vi "2013_02_18 Quality Main.vi"() -> ()   [LabVIEW 2013]
uses:
  Quality Type Def.ctl
  <vilib>/DAQmx/write.llb/DAQmx Write (Counter Time 1Chan 1Samp).vi
  <vilib>/DAQmx/read.llb/DAQmx Read (Analog 1D Wfm NChan NSamp).vi
  <vilib>/DAQmx/miscellaneous.llb/DAQmx Fill In Error Info.vi
  <resource>/objmgr/daqmx.rc
panel:
  out "Error":bool
  out "XY Graph 3":cluster{"Array":dbl[], "Array":dbl[]}[](graph)
  in  "X axis":u16(ring)=5 items=["Elapsed Time (s)"=0, "Source Current (A)"=10, "Supply (V)"=4, "Supply Power (W)"=11, "RMS Current (A) 1"=1, "RMS Voltage (V) 1"=2, "Electrical Power (W)"=6, "ESC Efficiency (%)"=12, "Torque (mNm)"=5, "RPM"=3, "Mechanical Power(W)"=7, "Motor Efficiency (%)"=8]
  in  "Capture":bool=TRUE
  in  "Y axis":u16(ring)=3 items=["Elapsed Time (s)"=0, "Source Current (A)"=10, "Supply (V)"=4, "Supply Power (W)"=11, "RMS Current (A) 1"=1, "RMS Voltage (V) 1"=2, "Electrical Power (W)"=6, "ESC Efficiency (%)"=12, "Torque (mNm)"=5, "RPM"=3, "Mechanical Power(W)"=7, "Motor Efficiency (%)"=8]
  out "TotalSampPerChanAcquired":dbl
  out "AvailSampPerChan":u32
  out "XY Graph 2":cluster{"Array":dbl[], "Array":dbl[]}[](graph)
  out "Single Motor 2":waveform(dbl)[](graph)
  in  "Waveform":bool
  out "XY Graph":cluster{"Array":dbl[], "Array":dbl[]}(graph)
  out "error out":errorcluster
  in  "File Path":path=path "C:/Users/Bullpen/Dropbox/Procyrion/Quality System/Hardware/Motors/Quality Results/.lvm"
  in  "Motor 1":T1 {"No Load Torque" format="%.3f"; "Stall Torque" format="%.3f"; "ESC Efficiency" format="%#_3g%%"; "Supply Power (W)" format="%.3f"; "Mechanical Power (W)" format="%.3f"; "Motor Efficiency" format="%#_3g%%"; "Electrical Power (W)" format="%.3f"; "Torque (mNm)" format="%.3f"; "Elapsed Time" format="%<%H:%M:%S>t"; "Supply (V)" format="%.2f"; "RPM" scale=0.0..60000.0}
  out "loop time (ms)":u32
  in  "stop":bool
  in  "PWM 1":dbl(slide) min=0.0 max=100.0 step=5.0 scale=0.0..100.0
  # "1. Run VI, drag \"PWM\" to 100%\n2. Enter serial and test description e.g. \"initial run\"\n3. Adjust supply voltage to desired no load speed\n4. Click \"Clear\" to clear graphs and data\n5. Load motor smoothly until stall, disable capture\n6. Enter no load speed, no load torque, stall torque\n7. Click \"Calculate\"\n8. Click \"Write\" when ready to save file (Desktop)\n9. Play with graphs"
  # "Fail"
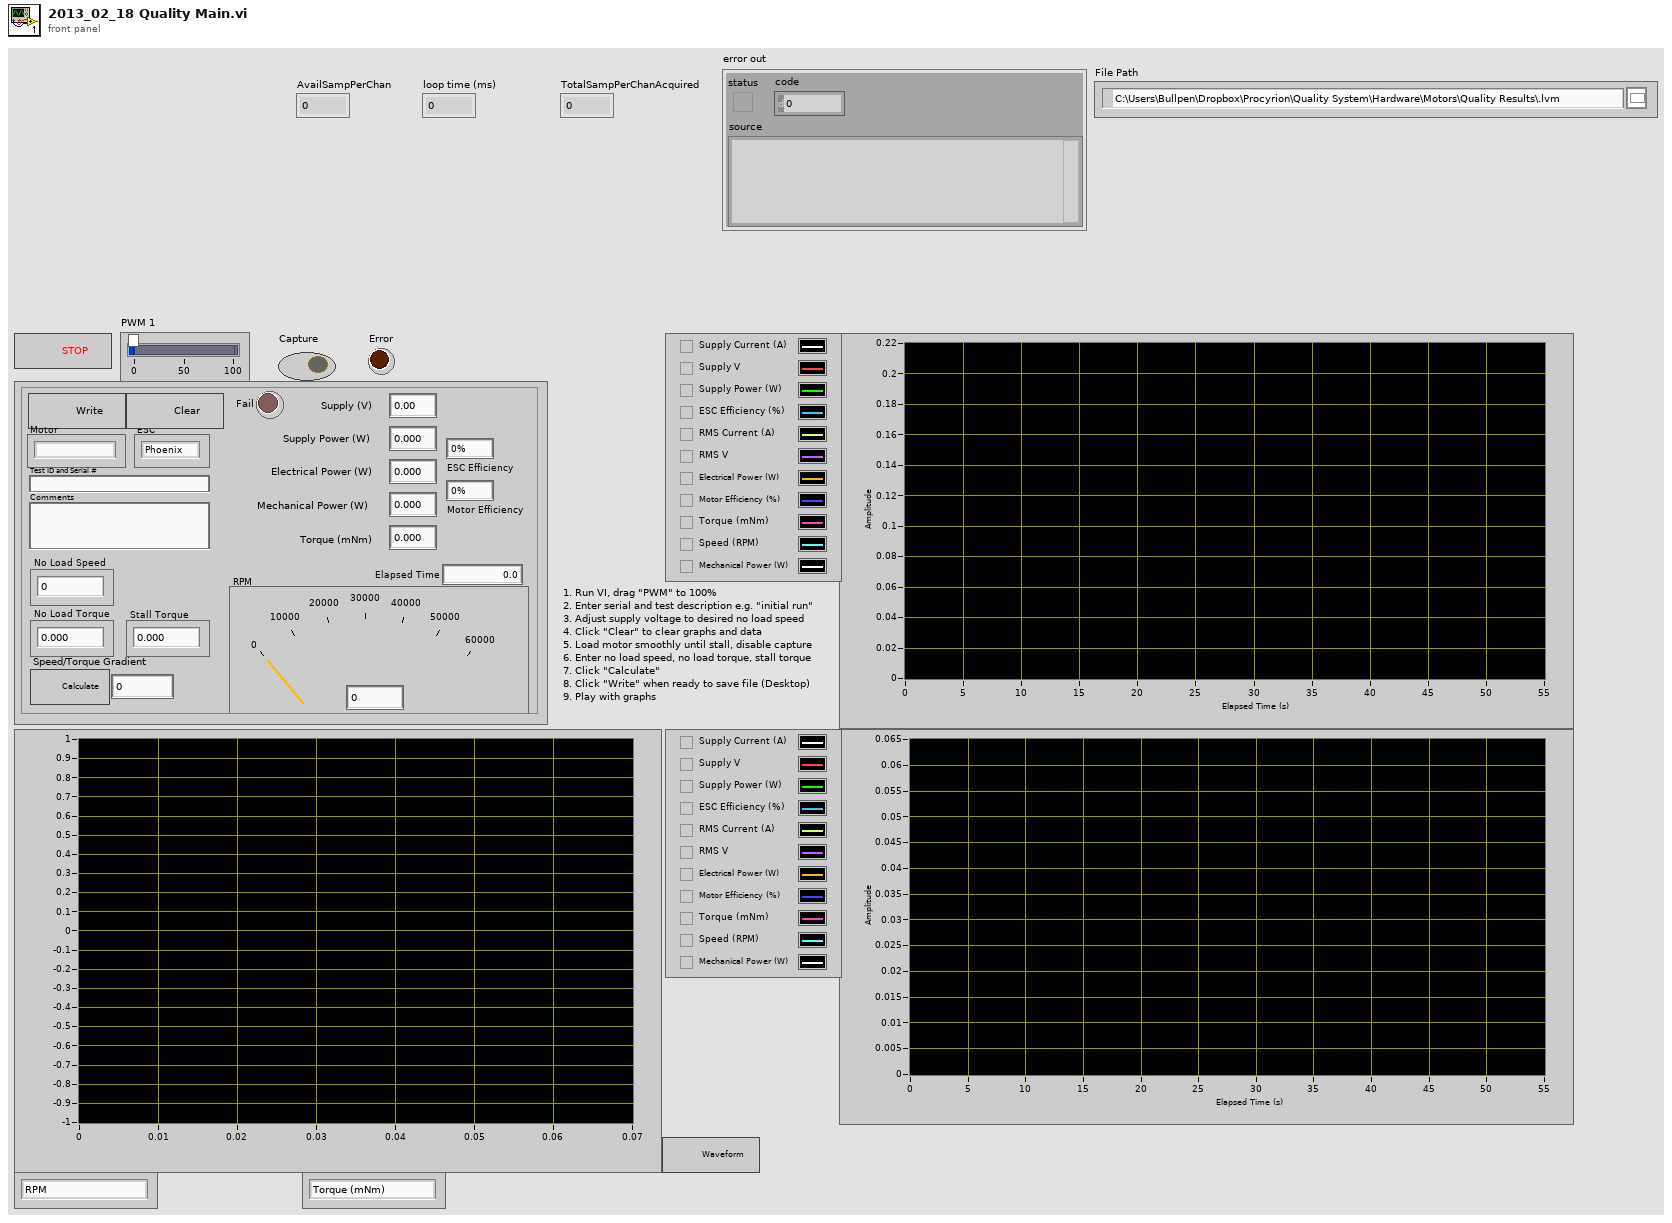
[diagram p1: front panel]
types:
  T1 = typedef "Quality Type Def.ctl" = cluster{"Write":bool, "Fail":bool, "RPM":u64, "Motor":enum16{"", "Maxon EC6 6V", "Maxon EC4 6V", "FH 0620 6V", "FH 0620 12V", "FH 0427 6V K2540"}, "ESC":enum16{"Phoenix", "Maxon", "FH 1801"}, "Supply (V)":dbl, "Test ID and Serial #":string, "Comments":string, "Elapsed Time":dbl, "Counter":dbl, "Torque (mNm)":dbl, "Electrical Power (W)":dbl, "Motor Efficiency":dbl, "Mechanical Power (W)":dbl, "Supply Power (W)":dbl, "ESC Efficiency":dbl, "No Load Speed":u32, "Stall Torque":dbl, "Speed/Torque Gradient":u32, "Calcul":bool, "Clear":bool, "No Load Torque":dbl}
  T2 = enum16{"", "Maxon EC6 6V", "Maxon EC4 6V", "FH 0620 6V", "FH 0620 12V", "FH 0427 6V K2540"}
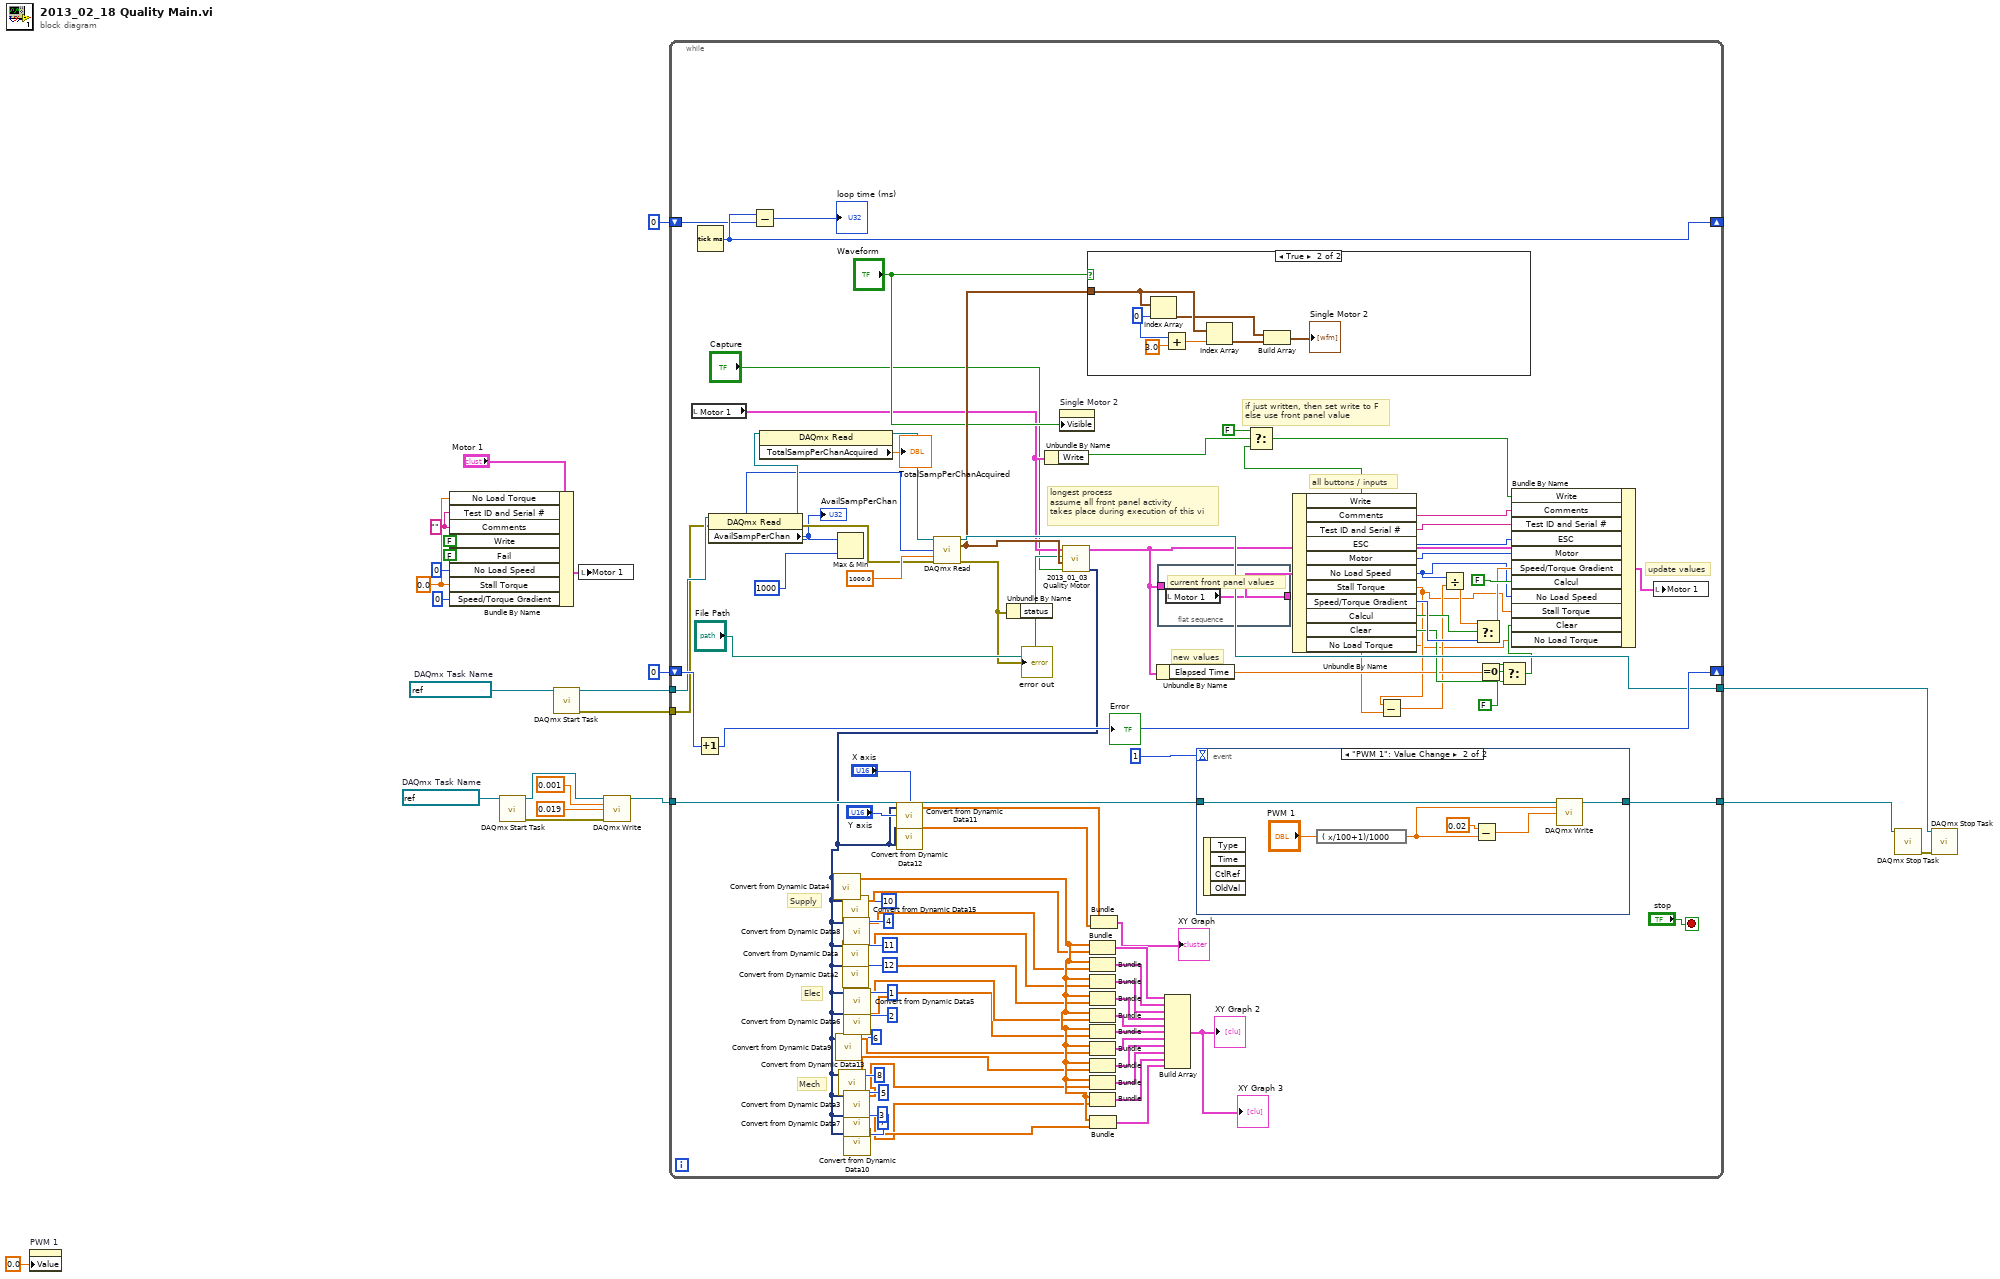
[diagram p0: block diagram]
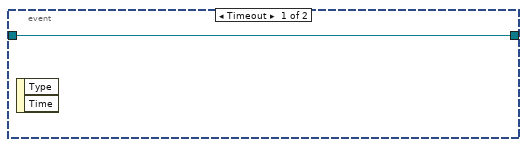
[diagram p3: hidden frame]
diagram:
  w3 = "" ("Comments")
  w2 = 0.0 ("Stall Torque")
  w21 = refnum<k21> "Flow PWM1"  # DAQmx Task Name
  w1 = refnum<k21> "Flow Acquire"  # DAQmx Task Name
  n1 = property on="PWM 1" class="Slide (strict)"("Value"=0.0 ("PWM 1")) -> ()  [unwired: 2 in, 2 out]
  n2 = Bundle By Name(cluster="Motor 1", "No Load Torque"=w2, "Test ID and Serial #"=w3, "Comments"=w3, "Write"=FALSE ("Enabled"), "Fail"=FALSE, "No Load Speed"=u32 0, "Stall Torque"=w2, "Speed/Torque Gradient"=u32 0) -> (w6:T1)
  n3 = call <vilib>:"DAQmx Start Task.vi"("task/channels in"=w21) -> ("task out"=w19:refnum<k21>, "error out"=w18:errorcluster)  [unwired: 13 in]
  n4 = call <vilib>:"DAQmx Start Task.vi"("task/channels in"=w1) -> ("task out"=w23:refnum<k21>, "error out"=w10:errorcluster)  [unwired: 13 in]
  n5 = local write "Motor 1"(w6) -> ()
  n6 = call-poly <vilib>:"DAQmx Write.vi"("task/channels in"=w19, "high time"=0.001 ("data"), "low time"=0.019 ("data"), "error in"=w18) -> ("task out"=w20:refnum<k21>)  [unwired: 9 in, 2 out]
  n7 = while {
    tunnel: w23 -> [w83]
    tunnel: [w106] -> w22
    tunnel: w10 -> [w81]
    shift-right: [w114] -> _
    shift-left: u32 0 ("millisecond timer value") -> [w113]
    tunnel: w20 -> [w111]
    tunnel: [w110] -> w17
    shift-right: [w107] -> _
    shift-left: 0 ("for") -> [w108]
    stop <- "stop" stop-if-true
    # "Mech"
    # "Elec"
    # "Supply"
    # "if just written, then set write to F\nelse use front panel value"
    # "all buttons / inputs"
    # "update values"
    # "new values"
    # "longest process\nassume all front panel activity\ntakes place during execution of this vi"
    n8 = local read "Motor 1"() -> (w58:T1)
    n9 = Increment(x=w108) -> (x+1=w107:i32)
    n10 = Tick Count (ms)() -> (millisecond timer value=w114:u32)
    n11 = property class="DAQmx Read"(reference=w83, error in=w81) -> (reference out=w79:refnum<k21>, error out=w80:errorcluster, "AvailSampPerChan"=w75:u32)
    "AvailSampPerChan" <- w75
    n12 = Subtract(x=w114, y=w113) -> (x-y=→"loop time (ms)":u32)
    n13 = property class="DAQmx Read"(reference=w79) -> (reference out=w78:refnum<k21>, "TotalSampPerChanAcquired"=→"TotalSampPerChanAcquired":dbl)  [unwired: 1 in, 1 out]
    n14 = Max & Min(x=w75, y=1000 ("number of samples per channel")) -> (max(x,y)=w74:u32)  [unwired: 1 out]
    n15 = call-poly <vilib>:"DAQmx Read.vi"("task/channels in"=w78, "number of samples per channel"=w74, "timeout"=1000.0, "error in"=w80) -> ("task out"=w106:refnum<k21>, "data"=w104:waveform(dbl)[], "error out"=w24:errorcluster)  [unwired: 9 in]
    "error out" <- w24
    n16 = Unbundle By Name(w24) -> ()  [unwired: 1 out]
    n17 = Unbundle By Name(w58) -> ("Write"=w57:bool)
    n18 = property on="Single Motor 2" class="WFGraph (strict)"("Visible"="Waveform") -> ()  [unwired: 2 in, 2 out]
    n19 = call "2013_01_03 Quality Motor.vi"("Capture"="Capture", "data"=w104, "File Path"="File Path", "Motor Typedef"=w58) -> ("Final Out"=w70:dynamicdata, "Motor Typedef Out"=w64:T1)  [unwired: 6 in]
    n20 = call "Convert from Dynamic Data4"("Dynamic Data Type"=w70) -> ("Array"=w50:dbl[])  [unwired: 3 in]
    n21 = call "Convert from Dynamic Data9"("Dynamic Data Type"=w70, "Channel"=6) -> ("Array"=w48:dbl[])  [unwired: 2 in]
    n22 = call "Convert from Dynamic Data13"("Dynamic Data Type"=w70, "Channel"=8) -> ("Array"=w26:dbl[])  [unwired: 2 in]
    n23 = call "Convert from Dynamic Data15"("Dynamic Data Type"=w70, "Channel"=10) -> ("Array"=w49:dbl[])  [unwired: 2 in]
    n24 = call "Convert from Dynamic Data"("Dynamic Data Type"=w70, "Channel"=11) -> ("Array"=w33:dbl[])  [unwired: 2 in]
    n25 = call "Convert from Dynamic Data2"("Dynamic Data Type"=w70, "Channel"=12) -> ("Array"=w32:dbl[])  [unwired: 2 in]
    n26 = call "Convert from Dynamic Data8"("Dynamic Data Type"=w70, "Channel"=4) -> ("Array"=w34:dbl[])  [unwired: 2 in]
    n27 = call "Convert from Dynamic Data3"("Dynamic Data Type"=w70, "Channel"=5) -> ("Array"=w27:dbl[])  [unwired: 2 in]
    n28 = call "Convert from Dynamic Data7"("Dynamic Data Type"=w70, "Channel"=3) -> ("Array"=w28:dbl[])  [unwired: 2 in]
    n29 = call "Convert from Dynamic Data5"("Dynamic Data Type"=w70, "Channel"=1) -> ("Array"=w31:dbl[])  [unwired: 2 in]
    n30 = call "Convert from Dynamic Data6"("Dynamic Data Type"=w70, "Channel"=2) -> ("Array"=w30:dbl[])  [unwired: 2 in]
    n31 = call "Convert from Dynamic Data10"("Dynamic Data Type"=w70, "Channel"=7) -> ("Array"=w29:dbl[])  [unwired: 2 in]
    n32 = call "Convert from Dynamic Data11"("Dynamic Data Type"=w70, "Channel"="X axis") -> ("Array"=w71:dbl[])  [unwired: 2 in]
    n33 = call "Convert from Dynamic Data12"("Dynamic Data Type"=w70, "Channel"="Y axis") -> ("Array"=w72:dbl[])  [unwired: 2 in]
    n34 = case shown="True" "Waveform" {
      tunnel: w104 -> [_ w121]
      frame False {
      }
      frame True {
        w122 = 0 ("index")
        n35 = Index Array(array=w121, index=w122) -> (element=w119:waveform(dbl))
        n36 = Add(x=w122, y=3.0) -> (x+y=w120:dbl)
        n37 = Index Array(array=w121, index=w120) -> (element=w118:waveform(dbl))
        n38 = Build Array(w119, w118) -> (→"Single Motor 2":waveform(dbl)[])
      }
    }
    n39 = Bundle("Array"=w50, "Array"=w49) -> (w93:cluster{"Array":dbl[], "Array":dbl[]})  [unwired: 1 in]
    n40 = Bundle("Array"=w50, "Array"=w34) -> (w94:cluster{"Array":dbl[], "Array":dbl[]})  [unwired: 1 in]
    n41 = Bundle("Array"=w50, "Array"=w33) -> (w95:cluster{"Array":dbl[], "Array":dbl[]})  [unwired: 1 in]
    n42 = Bundle("Array"=w50, "Array"=w32) -> (w96:cluster{"Array":dbl[], "Array":dbl[]})  [unwired: 1 in]
    n43 = Bundle("Array"=w50, "Array"=w31) -> (w97:cluster{"Array":dbl[], "Array":dbl[]})  [unwired: 1 in]
    n44 = Bundle("Array"=w50, "Array"=w30) -> (w98:cluster{"Array":dbl[], "Array":dbl[]})  [unwired: 1 in]
    n45 = Bundle("Array"=w50, "Array"=w48) -> (w99:cluster{"Array":dbl[], "Array":dbl[]})  [unwired: 1 in]
    n46 = Bundle("Array"=w50, "Array"=w26) -> (w100:cluster{"Array":dbl[], "Array":dbl[]})  [unwired: 1 in]
    n47 = Bundle("Array"=w50, "Array"=w27) -> (w102:cluster{"Array":dbl[], "Array":dbl[]})  [unwired: 1 in]
    n48 = Bundle("Array"=w50, "Array"=w28) -> (w101:cluster{"Array":dbl[], "Array":dbl[]})  [unwired: 1 in]
    n49 = Bundle("Array"=w50, "Array"=w29) -> (w91:cluster{"Array":dbl[], "Array":dbl[]})  [unwired: 1 in]
    n50 = Bundle("Array"=w71, "Array"=w72) -> (→"XY Graph":cluster{"Array":dbl[], "Array":dbl[]})  [unwired: 1 in]
    n51 = Unbundle By Name(w64) -> ("Elapsed Time"=w65:dbl)
    n52 = flat-sequence {
      tunnel: w64 -> [_]
      tunnel: [w116] -> w63
      frame #0 {
        # "current front panel values"
        n53 = local read "Motor 1"() -> (w116:T1)
      }
    }
    n54 = Build Array(w93, w94, w95, w96, w97, w98, w99, w100, w102, w101, w91) -> (→"XY Graph 2" →"XY Graph 3":cluster{"Array":dbl[], "Array":dbl[]}[])
    n55 = event shown="[1] \"PWM 1\": Value Change" {
      selector: _ -> [_ _]
      dyn-events: _ -> [_ _]
      timeout: 1 -> [_ _]
      tunnel: w111 -> [w124 w126]
      tunnel: [w124 w125] -> w110
      event Timeout {
        n56 = event-data() -> ()  [unwired: 1 in, 2 out]
      }
      event "PWM 1": Value Change {
        n57 = event-data() -> ()  [unwired: 1 in, 4 out]
        n58 = expression code="( x/100+1)/1000"("PWM 1") -> (w127:dbl)
        n59 = Subtract(x=0.02 ("y"), y=w127) -> (x-y=w128:dbl)
        n60 = call-poly <vilib>:"DAQmx Write.vi"("task/channels in"=w126, "high time"=w127, "low time"=w128) -> ("task out"=w125:refnum<k21>)  [unwired: 10 in, 2 out]
      }
    }
    n61 = Unbundle By Name(w63) -> ("Write"=w55:bool, "Comments"=w62:string, "Test ID and Serial #"=w61:string, "ESC"=w60:enum16{"Phoenix", "Maxon", "FH 1801"}, "Motor"=w59:T2, "No Load Speed"=w85:u32, "Stall Torque"=w52:dbl, "Speed/Torque Gradient"=w87:u32, "Calcul"=w86:bool, "Clear"=w67:bool, "No Load Torque"=w51:dbl)
    n62 = Select(t=FALSE, s=w57, f=w55) -> (s? t:f=w54:bool)
    n63 = Subtract(x=w52, y=w51) -> (x-y=w53:dbl)
    n64 = Divide(x=w85, y=w53) -> (x/y=w89:dbl)
    n65 = Select(t=w89, s=w86, f=w87) -> (s? t:f=w88:dbl)
    n66 = Equal To 0?(x=w65) -> (x = 0?=w69:bool)
    n67 = Select(t=FALSE ("Calcul"), s=w69, f=w67) -> (s? t:f=w66:bool)
    n68 = Bundle By Name(cluster=w64, "Write"=w54, "Comments"=w62, "Test ID and Serial #"=w61, "ESC"=w60, "Motor"=w59, "Speed/Torque Gradient"=w88, "Calcul"=FALSE, "No Load Speed"=w85, "Stall Torque"=w52, "Clear"=w66, "No Load Torque"=w51) -> (w105:T1)
    n69 = local write "Motor 1"(w105) -> ()
  }
  n70 = call <vilib>:"DAQmx Stop Task.vi"("task/channels in"=w17) -> ("error out"=w16:errorcluster)  [unwired: 13 in, 1 out]
  n71 = call <vilib>:"DAQmx Stop Task.vi"("task/channels in"=w22, "error in"=w16) -> ()  [unwired: 12 in, 2 out]
